vi "Set Top Level Library.vi"(8 "error in (no error)":errorcluster, 10 "ProjectItem Refnum":refnum<vi>, 11 "PPL in":refnum<class "NI_AB_API_DPPL.lvclass">) -> (0 "error out":errorcluster, 3 "PPL out":refnum<class "NI_AB_API_DPPL.lvclass">)   [LabVIEW 2020, in "NI_AB_API_DPPL.lvclass"]
uses:
  <vilib>/AppBuilder/AB_API/DPPL/NI_AB_API_DPPL.lvclass
  <vilib>/AppBuilder/AB_API/PPL/NI_AB_API_PPL.lvclass
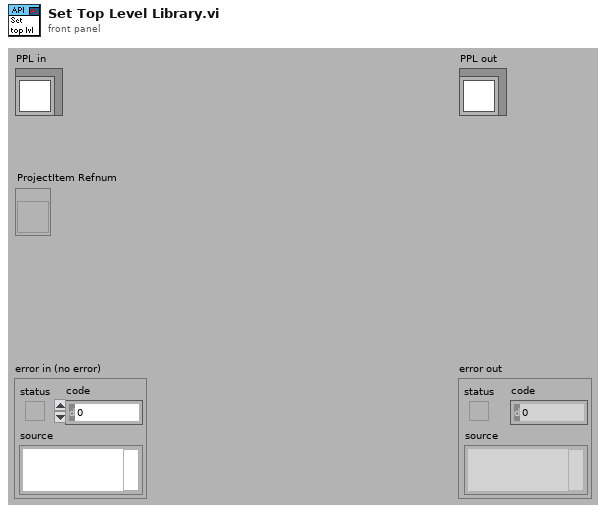
[diagram p1: front panel]
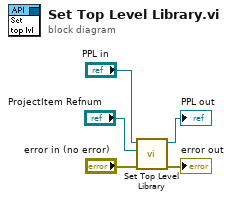
[diagram p0: block diagram]
diagram:
  n1 = call-parent "Set Top Level Library.vi"("error in (no error)"="error in (no error)", "ProjectItem Refnum"="ProjectItem Refnum", "PPL in"="PPL in") -> ("error out"=→"error out":errorcluster, "PPL out"=→"PPL out":refnum<class "NI_AB_API_DPPL.lvclass">)  [unwired: 7 in]
